vi "_isBufferEmpty.vi"(11 "VariantBuffer in":refnum<class "VariantBuffer.lvclass">) -> (2 "isEmpty":bool)   [LabVIEW 2013, in "CircularBuffer.lvlib" / "VariantBuffer.lvclass"]
uses:
  VariantBuffer.lvclass
  VariantBuffer.lvclass/VariantBuffer.ctl
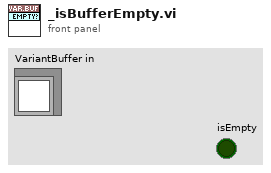
[diagram p1: front panel]
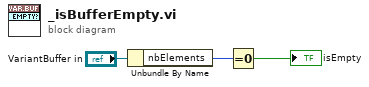
[diagram p0: block diagram]
diagram:
  n1 = Unbundle By Name("VariantBuffer in") -> ("nbElements"=w2:i32)
  n2 = Equal To 0?(x=w2) -> (x = 0?=→"isEmpty":bool)
